vi "ReadSetting.vi"(0 "Data Filename":string) -> (1 "Phase":dbl=7.3 format="%#_13g", 2 "Tune":dbl=2.321 format="%#_13g", 3 "File path":string="C:\\Users\\plm\\Desktop\\rssmt\\data\\TEQ3559748002.csv")   [LabVIEW 2018]
uses:
  <vilib>/Utility/file.llb/Read From Spreadsheet File (string).vi
  <vilib>/Utility/file.llb/Read From Spreadsheet File (DBL).vi
  Global 2.vi
panel:
  out "IF/Log":dbl=2.0 format="%#_13g"
  out "Invert":dbl=2.0 format="%#_13g"
  out "Gain":dbl=2.0 format="%#_13g"
  out "IFatt dB":dbl=10.0 format="%#_13g"
  out "RFgen dBm":dbl=9.0 format="%#_13g"
  out "Chan #":dbl=2.0 format="%#_13g"
  out "Qamp":dbl=1.7 format="%#_13g"
  out "Offset":dbl=3.9884 format="%#_13g"
  out "Nstep":dbl=201.0 format="%#_13g"
  out "Fstep":dbl=0.001 format="%#_13g"
  out "Array Vals":dbl[](array[numeric])=[35597.0, 48002.8979, 224.47, 0.001, 201.0, 1.0, 25.75, 3.294, 2.321, 3.9884, 7.3, 3.9795, 1.7, 1.0, 2.0, 1.0, 0.0, 0.1642, 2.0, 224.4705, 0.0, 9.0, 10.0, 0.0, 0.0]
  out "Array":dbl[][](array[numeric])=[[213.0, 0.0], [0.0, 0.0], [0.0, 0.0], [0.0, 0.0], [0.0, 0.0], [0.0, 0.0], [0.0, 0.0], [0.0, 0.0], [0.0, 0.0], [0.0, 0.0], [35597.0, 0.0], [48002.8979, 0.0], [224.47, 0.0], [0.001, 0.0], [201.0, 0.0], [1.0, 0.0], [25.75, 0.0], [3.294, 0.0], [2.321, 0.0], [3.9884, 0.0], [7.3, 0.0], [3.9795, 0.0], [1.7, 0.0], [1.0, 0.0], [2.0, 0.0], [1.0, 0.0], [0.0, 0.0], [0.1642, 0.0], [2.0, 0.0], [224.4705, 0.0], [0.0, 0.0], [9.0, 0.0], [10.0, 0.0], [0.0, 0.0], [0.0, 0.0]]
  out "Text":string[][](array[string])=[["213 MHz crystal", " SMT03 RF Gen"], ["NMRave.xls", ""], ["Unused", ""], ["NMRave.xls", ""], ["Unused", ""]]
  out "Chars":i32=381
  out "Fcen":dbl=224.47 format="%#_13g"
  out "File size (bytes)":i32=2793000
  # "Loader for global NMR Settings"
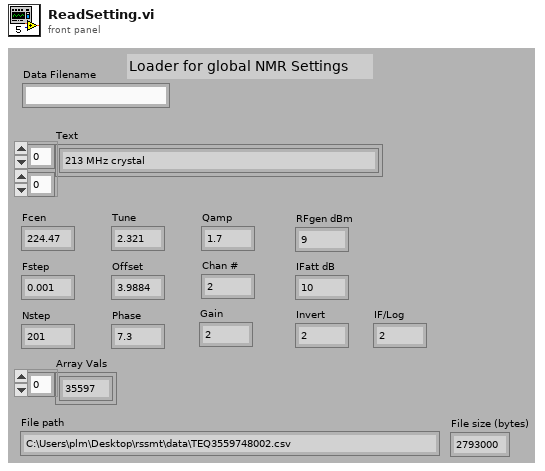
[diagram p1: front panel]
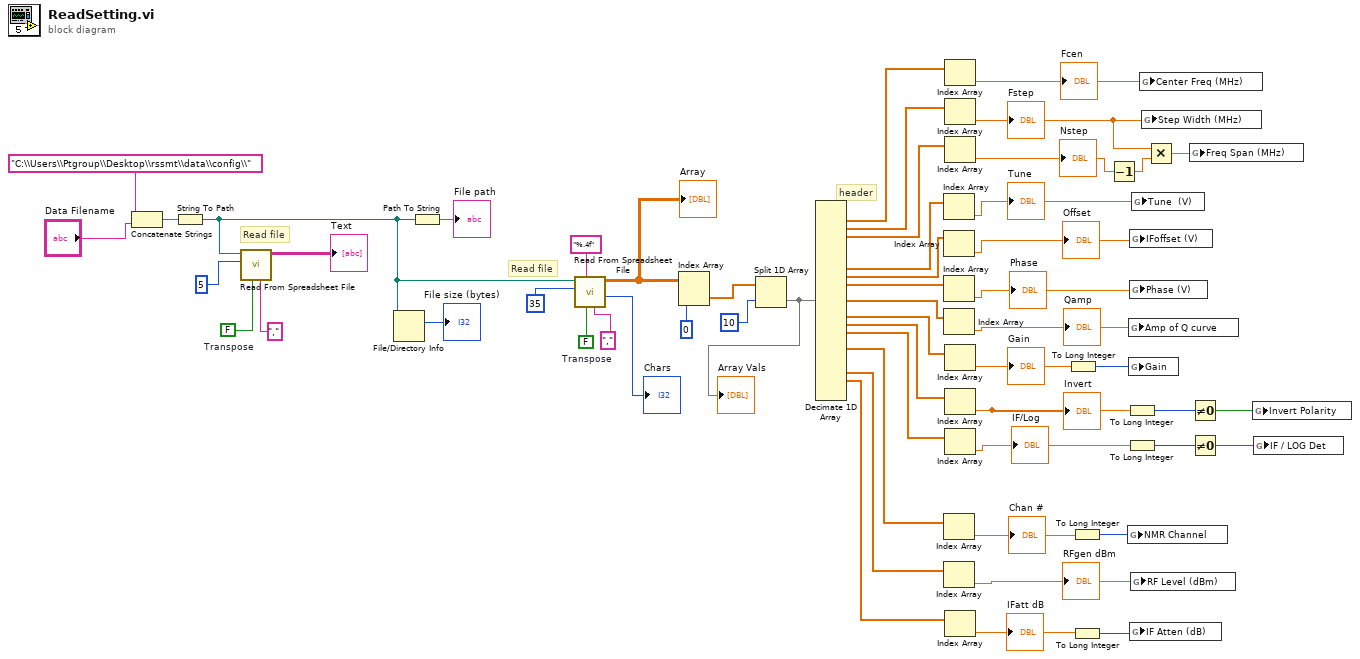
[diagram p0: block diagram]
diagram:
  w42 = FALSE  # Transpose
  w52 = FALSE  # Transpose
  # "Read file"
  # "Read file"
  # "header"
  n1 = Concatenate Strings "Concatenate Strings"("C:\\Users\\Ptgroup\\Desktop\\rssmt\\data\\config\\", "Data Filename") -> (w54:string)
  n2 = String To Path(string=w54) -> (path=w44:path)
  n3 = call-poly <vilib>:"Read From Spreadsheet File.vi"("delimiter (\\t)"=",", "transpose (no:F)"=w42, "number of rows (all:-1)"=5, "file path (dialog if empty)"=w44) -> ("all rows"=→"Text":string[][])  [unwired: 3 in, 4 out]
  n4 = File/Directory Info(path=w44) -> (size=→"File size (bytes)":i64)  [unwired: 1 in, 6 out]
  n5 = Path To String(path=w44) -> (string=→"File path":string)
  n6 = call-poly <vilib>:"Read From Spreadsheet File.vi"("delimiter (\\t)"=",", "transpose (no:F)"=w52, "format (%.3f)"="%.4f", "number of rows (all:-1)"=35, "file path (dialog if empty)"=w44) -> ("mark after read (chars.)"=→"Chars":i32, "all rows"=w37:dbl[][])  [unwired: 2 in, 3 out]
  "Array" <- w37
  n7 = Index Array "Index Array"(array=w37, index (col)=0) -> (element=w36:dbl[])  [unwired: 1 in]
  n8 = Split 1D Array(array=w36, index=10) -> (second subarray=w34:dbl[])  [unwired: 1 out]
  "Array Vals" <- w34
  n9 = Decimate 1D Array(w34) -> (w48:dbl[], w47:dbl[], w46:dbl[], w33:dbl[], w32:dbl[], w31:dbl[], w30:dbl[], w26:dbl[], w8:dbl[], w7:dbl[], w29:dbl[], w28:dbl[], w27:dbl[])  [unwired: 12 out]
  n10 = Index Array(array=w33) -> (element=w25:dbl)  [unwired: 1 in]
  "Tune" <- w25
  n11 = Index Array(array=w32) -> (element=w24:dbl)  [unwired: 1 in]
  "Offset" <- w24
  n12 = Index Array(array=w31) -> (element=w23:dbl)  [unwired: 1 in]
  "Phase" <- w23
  n13 = Index Array(array=w30) -> (element=w22:dbl)  [unwired: 1 in]
  "Qamp" <- w22
  n14 = Index Array(array=w29) -> (element=w21:dbl)  [unwired: 1 in]
  "Chan #" <- w21
  n15 = Index Array(array=w28) -> (element=w11:dbl)  [unwired: 1 in]
  "RFgen dBm" <- w11
  n16 = Index Array "Index Array"(array=w48) -> (element=w19:dbl)  [unwired: 1 in]
  "Fcen" <- w19
  n17 = Index Array(array=w47) -> (element=w18:dbl)  [unwired: 1 in]
  "Fstep" <- w18
  n18 = Index Array(array=w46) -> (element=w17:dbl)  [unwired: 1 in]
  "Nstep" <- w17
  n19 = Index Array(array=w26) -> (element=w10:dbl)  [unwired: 1 in]
  "Gain" <- w10
  n20 = Index Array(array=w8) -> (element=w5:dbl)  [unwired: 1 in]
  "Invert" <- w5
  n21 = Index Array(array=w7) -> (element=w6:dbl)  [unwired: 1 in]
  "IF/Log" <- w6
  n22 = Index Array(array=w27) -> (element=w13:dbl)  [unwired: 1 in]
  "IFatt dB" <- w13
  n23 = To Long Integer(number=w10) -> (32bit integer=w9:i32)
  n24 = To Long Integer(number=w21) -> (32bit integer=w20:i32)
  n25 = To Long Integer(number=w13) -> (32bit integer=w12:i32)
  n26 = Decrement(x=w17) -> (x-1=w16:dbl)
  n27 = To Long Integer(number=w5) -> (32bit integer=w4:i32)
  n28 = To Long Integer(number=w6) -> (32bit integer=w3:i32)
  n29 = global write "Global 2.vi" "NMR Channel"(w20) -> ()
  n30 = global write "Global 2.vi" "Amp of Q curve"(w22) -> ()
  n31 = global write "Global 2.vi" "Gain"(w9) -> ()
  n32 = global write "Global 2.vi" "IFoffset (V)"(w24) -> ()
  n33 = global write "Global 2.vi" "Phase (V)"(w23) -> ()
  n34 = global write "Global 2.vi" "IF Atten (dB)"(w12) -> ()
  n35 = global write "Global 2.vi" "RF Level (dBm)"(w11) -> ()
  n36 = global write "Global 2.vi" "Tune  (V)"(w25) -> ()
  n37 = global write "Global 2.vi" "Center Freq (MHz)"(w19) -> ()
  n38 = global write "Global 2.vi" "Step Width (MHz)"(w18) -> ()
  n39 = Multiply(x=w18, y=w16) -> (x*y=w15:dbl)
  n40 = global write "Global 2.vi" "Freq Span (MHz)"(w15) -> ()
  n41 = Not Equal To 0?(x=w4) -> (x != 0?=w2:bool)
  n42 = Not Equal To 0?(x=w3) -> (x != 0?=w1:bool)
  n43 = global write "Global 2.vi" "Invert Polarity"(w2) -> ()
  n44 = global write "Global 2.vi" "IF / LOG Det"(w1) -> ()
